vi "Support releaseFileEOF.vi"(8 "error in (no error)":errorcluster) -> (0 "error out":errorcluster)   [LabVIEW 2018]
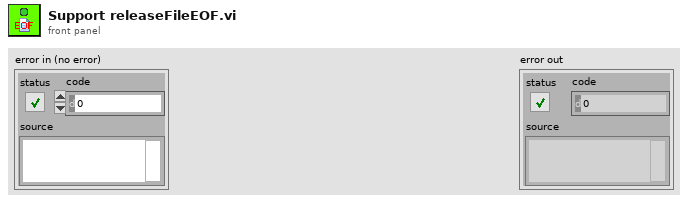
[diagram p1: front panel]
types:
  T1 = enum16{"open", "replace", "create", "open or create", "replace or create", "replace or create with confirmation"}
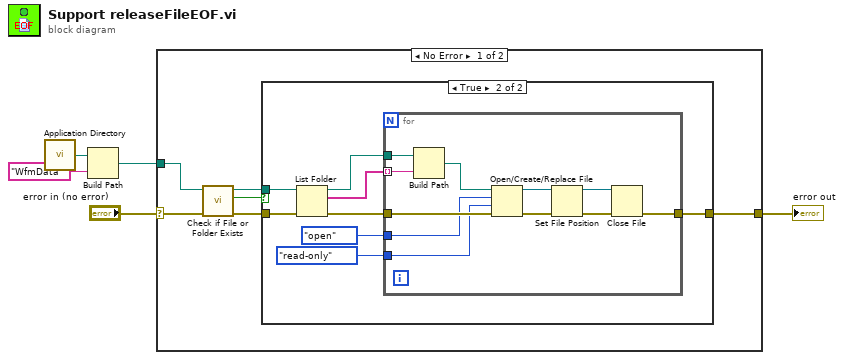
[diagram p0: block diagram]
diagram:
  n1 = call <vilib>:"Application Directory.vi"() -> ("Application Directory"=w5:path)
  n2 = Build Path(base path=w5, name or relative path="WfmData") -> (appended path=w3:path)
  n3 = case shown="No Error" "error in (no error)" {
    selector: "error in (no error)" -> [w7 w32]
    tunnel: w3 -> [w6 _]
    tunnel: [w8 w32] -> w2
    frame No Error {
      n4 = call <vilib>:"Check if File or Folder Exists.vi"("error in (no error)"=w7, "path"=w6) -> ("error out"=w10:errorcluster, "file or folder exists?"=w11:bool, "dup path"=w9:path)  [unwired: 7 in]
      n5 = case shown="True" w11 {
        tunnel: w10 -> [w12 w19]
        tunnel: w9 -> [_ w20]
        tunnel: [w12 w13] -> w8
        frame False {
        }
        frame True {
          n6 = List Folder(path=w20, error in=w19) -> (path out=w16:path, filenames=w17:string[], error out=w18:errorcluster)  [unwired: 2 in, 1 out]
          n7 = for {
            tunnel: w18 -> [w28]
            tunnel: w17 -> [w31] mode=indexing
            tunnel: w16 -> [w30]
            tunnel: T1."open" ("operation (0:open)") -> [w27]
            tunnel: enum16{"read/write", "read-only", "write-only"}."read-only" ("access (0:read/write)") -> [w26]
            tunnel: [w21] -> w13
            n8 = Build Path(base path=w30, name or relative path=w31) -> (appended path=w29:path)
            n9 = Open/Create/Replace File(file path (use dialog)=w29, error in=w28, operation (0:open)=w27, access (0:read/write)=w26) -> (refnum out=w25:refnum<file>, error out=w24:errorcluster)  [unwired: 2 in, 1 out]
            n10 = Set File Position(refnum=w25, error in=w24) -> (refnum out=w23:refnum<file>, error out=w22:errorcluster)  [unwired: 2 in]
            n11 = Close File(refnum=w23, error in=w22) -> (error out=w21:errorcluster)  [unwired: 1 out]
          }
        }
      }
    }
    frame Error {
    }
  }
  "error out" <- w2
